vi "Electronic Procedure.vi"() -> ()   [LabVIEW 2017]
panel:
  in  "Skip Step":bool
  out "Task Tip":string
  out "Experiment Progress":dbl(slide) max=27.0 scale=0.0..3.0
  in  "?":bool
  out "Task 5":bool caption="Set pump frequency"
  out "Task 4":bool caption="Set pump frequency"
  out "Task 3":bool caption="Set pump frequency"
  out "Task 1":bool caption="Start Action Table"
  out "Task 2":bool caption="Reactor Operator"
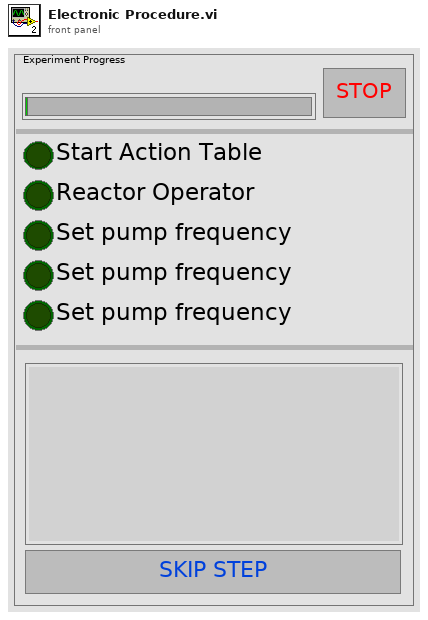
[diagram p1: front panel]
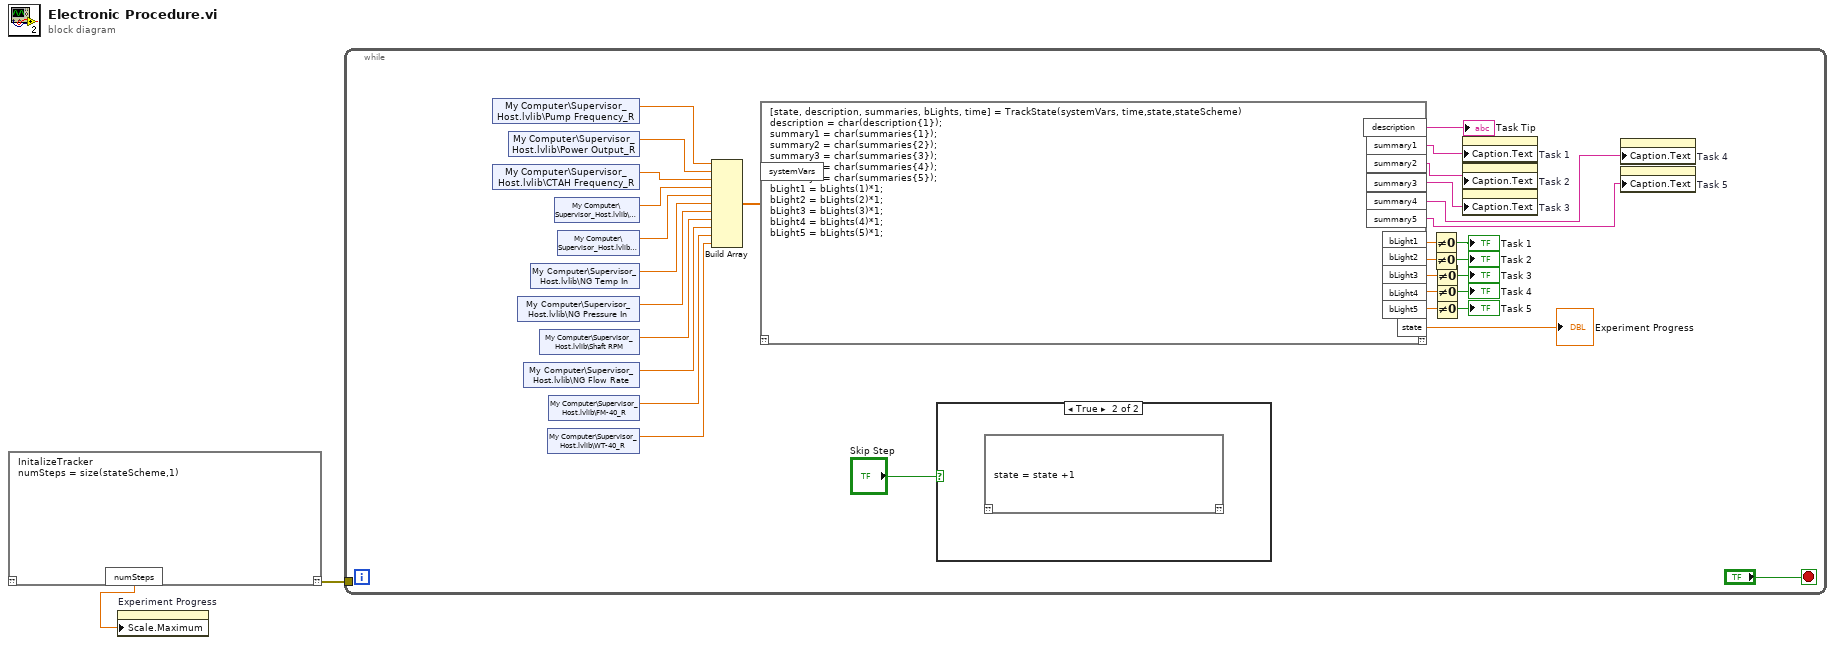
[diagram p0: block diagram]
diagram:
  n1 = script code="InitalizeTracker\nnumSteps = size(stateScheme,1)"() -> ("??"=w2:errorcluster, "numSteps"=w1:dbl)  [unwired: 1 in]
  n2 = property on="Experiment Progress" class="Slide (strict)"("Scale.Maximum"=w1) -> ()  [unwired: 2 in, 2 out]
  n3 = while {
    tunnel: w2 -> [_]
    stop <- "?" stop-if-true
    n4 = shared-variable "My Computer\\Supervisor_Host.lvlib\\Pump Frequency_R"() -> (w14:sgl)  [unwired: 1 in, 1 out]
    n5 = shared-variable "My Computer\\Supervisor_Host.lvlib\\CTAH Frequency_R"() -> (w12:sgl)  [unwired: 1 in, 1 out]
    n6 = shared-variable "My Computer\\Supervisor_Host.lvlib\\Power Output_R"() -> (w13:sgl)  [unwired: 1 in, 1 out]
    n7 = shared-variable "My Computer\\Supervisor_Host.lvlib\\NG Pressure In"() -> (w8:sgl)  [unwired: 1 in, 1 out]
    n8 = shared-variable "My Computer\\Supervisor_Host.lvlib\\NG Flow Rate"() -> (w6:sgl)  [unwired: 1 in, 1 out]
    n9 = shared-variable "My Computer\\Supervisor_Host.lvlib\\NG Temp In"() -> (w9:sgl)  [unwired: 1 in, 1 out]
    n10 = shared-variable "My Computer\\Supervisor_Host.lvlib\\Shaft RPM"() -> (w7:sgl)  [unwired: 1 in, 1 out]
    n11 = shared-variable "My Computer\\Supervisor_Host.lvlib\\WT-40_R"() -> (w4:sgl)  [unwired: 1 in, 1 out]
    n12 = shared-variable "My Computer\\Supervisor_Host.lvlib\\FM-40_R"() -> (w5:sgl)  [unwired: 1 in, 1 out]
    n13 = shared-variable "My Computer\\Supervisor_Host.lvlib\\HPT PR"() -> (w11:sgl)  [unwired: 1 in, 1 out]
    n14 = shared-variable "My Computer\\Supervisor_Host.lvlib\\LPT PR"() -> (w10:sgl)  [unwired: 1 in, 1 out]
    n15 = Build Array(w14, w13, w12, w11, w10, w9, w8, w7, w6, w5, w4) -> (w15:sgl[])
    n16 = script code="[state, description, summaries, bLights, time] = TrackState(systemVars, time,state,stateScheme)\ndescription = char(description{1});\nsummary1 = char(summaries{1});\nsummary2 = char(summaries{2});\nsummary3 = char(summaries{3});\nsummary4 = char(summaries{4});\nsummary5 = char(summaries{5}); \nbLight1 = bLights(1)*1;\nbLight2 = bLights(2)*1;\nbLight3 = bLights(3)*1;\nbLight4 = bLights(4)*1;\nbLight5 = bLights(5)*1;"("systemVars"=w15) -> ("description"=→"Task Tip":string, "summary1"=w20:string, "summary2"=w19:string, "summary3"=w18:string, "summary4"=w17:string, "summary5"=w16:string, "bLight1"=w33:dbl, "bLight2"=w31:dbl, "bLight3"=w28:dbl, "bLight4"=w27:dbl, "bLight5"=w26:dbl, "state"=→"Experiment Progress":dbl)  [unwired: 1 in, 1 out]
    n17 = case shown="True" "Skip Step" {
      frame False {
      }
      frame True {
        n18 = script code="state = state +1"() -> ()  [unwired: 1 in, 1 out]
      }
    }
    n19 = Not Equal To 0?(x=w33) -> (x != 0?=→"Task 1":bool)
    n20 = Not Equal To 0?(x=w31) -> (x != 0?=→"Task 2":bool)
    n21 = Not Equal To 0?(x=w28) -> (x != 0?=→"Task 3":bool)
    n22 = Not Equal To 0?(x=w27) -> (x != 0?=→"Task 4":bool)
    n23 = Not Equal To 0?(x=w26) -> (x != 0?=→"Task 5":bool)
    n24 = property on="Task 1" class="Bool (strict)"("Caption.Text"=w20) -> ()  [unwired: 2 in, 2 out]
    n25 = property on="Task 2" class="Bool (strict)"("Caption.Text"=w19) -> ()  [unwired: 2 in, 2 out]
    n26 = property on="Task 3" class="Bool (strict)"("Caption.Text"=w18) -> ()  [unwired: 2 in, 2 out]
    n27 = property on="Task 4" class="Bool (strict)"("Caption.Text"=w17) -> ()  [unwired: 2 in, 2 out]
    n28 = property on="Task 5" class="Bool (strict)"("Caption.Text"=w16) -> ()  [unwired: 2 in, 2 out]
  }
